vi "Get Calibration from Selected File.vi"(11 "Calibration File":path) -> (3 "Slope":string)   [LabVIEW 2018, in "Pump Module.lvlib"]
uses:
  Pump Module.lvlib
  <vilib>/Utility/file.llb/Read Delimited Spreadsheet (string).vi
panel:
  out "size(s) 2":i32[](array[numeric])
  out "Last Row index":i32
  out "Last Row":string[](array[string])
  out "Full File":string[][](array[string])
  # "The 4th Column in the last row"
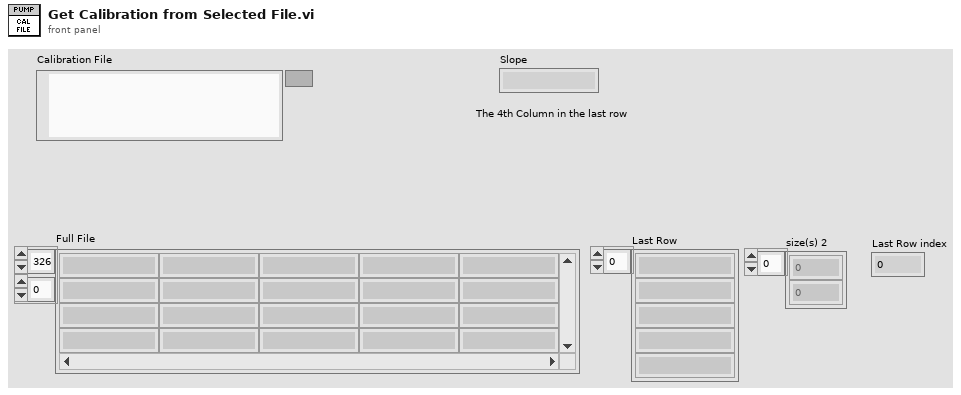
[diagram p1: front panel]
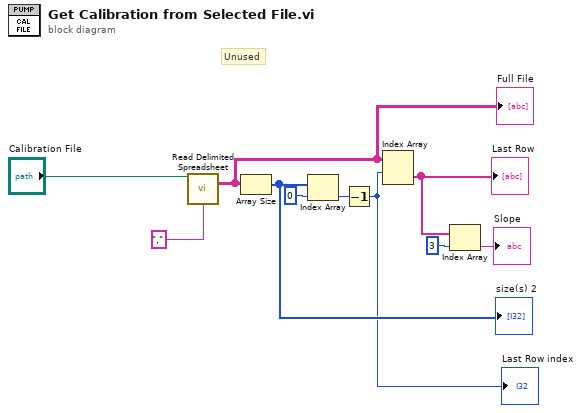
[diagram p0: block diagram]
diagram:
  # "Unused"
  n1 = call-poly <vilib>:"Read Delimited Spreadsheet.vi"("file path (dialog if empty)"="Calibration File", "delimiter (\\t)"="," ("delimiter (\\t)")) -> ("all rows"=w9:string[][])  [unwired: 8 in, 5 out]
  "Full File" <- w9
  n2 = Array Size(array=w9) -> (size(s)=w7:i32[])
  "size(s) 2" <- w7
  n3 = Index Array(array=w7, index=0) -> (element=w5:i32)
  n4 = Decrement(x=w5) -> (x-1=w4:i32)
  "Last Row index" <- w4
  n5 = Index Array(array=w9, index (row)=w4) -> (element=w2:string[])  [unwired: 1 in]
  "Last Row" <- w2
  n6 = Index Array(array=w2, index=3) -> (element=→"Slope":string)
